vi "Init VI.vi"(8 "error in (no error)":errorcluster, 10 "VI Refnum":refnum<vi>, 11 "Class in":refnum<class>) -> (0 "error out":errorcluster, 3 "Class out":refnum<class>)   [LabVIEW 2023, in "Label-Driven UI.lvlib"]
uses:
  Label-Driven UI.lvlib
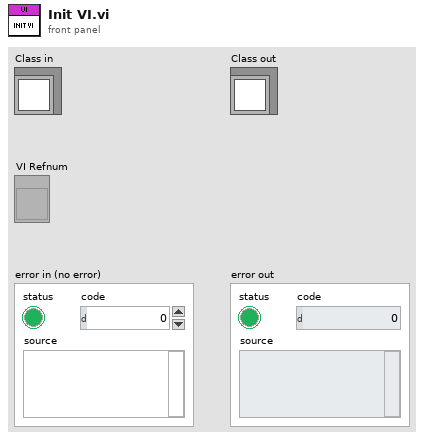
[diagram p1: front panel]
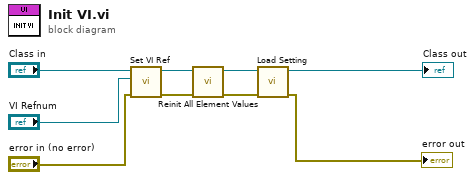
[diagram p0: block diagram]
diagram:
  n1 = call "Set VI Ref.vi"("error in"="error in (no error)", "VI Refnum"="VI Refnum", "Class in"="Class in") -> ("error out"=w6:errorcluster, "Class out"=w1:refnum<class>)  [unwired: 7 in]
  n2 = call "Reinit All Element Values.vi"("error in"=w6, "Class in"=w1) -> ("error out"=w7:errorcluster, "Class out"=w2:refnum<class>)  [unwired: 8 in]
  n3 = call "Load Setting.vi"("error in"=w7, "Class in"=w2) -> ("error out"=→"error out":errorcluster, "Class out"=→"Class out":refnum<class>)  [unwired: 8 in]
